vi "blob read.vi"(7 "iOffset":i32, 8 "error in (no error)":errorcluster, 9 "N":i32, 10 "Z":u32, 11 "para0":dbl) -> (0 "error out":errorcluster, 1 "function return":i32, 2 "Z out":u32, 3 "para0 out":dbl)   [LabVIEW 2020, in "sqlite3.lvlib"]
uses:
  sqlite3.lvlib
  errstr.vi
  bin/sqlite3_64.dll
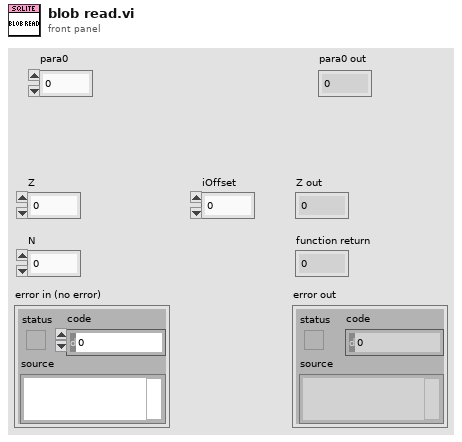
[diagram p1: front panel]
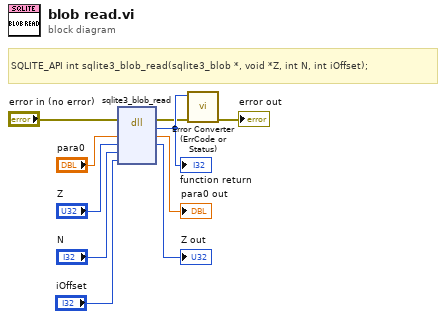
[diagram p0: block diagram]
diagram:
  # "SQLITE_API int sqlite3_blob_read(sqlite3_blob *, void *Z, int N, int iOffset);"
  n1 = dll-call lib="C:/Users/Fred.Guo/Desktop/Database-configuration/externals/sqlite3/Source/bin/sqlite3_*.*" fn="sqlite3_blob_read"(error in="error in (no error)", "para0"="para0", "Z"="Z", "N"="N", "iOffset"="iOffset") -> (error out=w2:errorcluster, w10:i32, "para0"=→"para0 out":dbl, "Z"=→"Z out":u32)  [unwired: 4 in, 1 out]
  "function return" <- w10
  n2 = call "Error Converter (ErrCode or Status).vi"("error in (no error)"=w2, "error code"=w10) -> ("error out"=→"error out":errorcluster)  [unwired: 9 in]
